vi "CRM-Config.vi"(6 "AI Channels":i32[](array[numeric]), 7 "Path":path, 8 "error in (no error)":errorcluster, 9 "Device Config":T1, 10 "Num AI pts":i32, 11 "Sampling Rate (Hz)":dbl=20000.0) -> (0 "error out":errorcluster, 1 "Magnitude array":dbl[](array[numeric]), 3 "Freq resol (Hz)":dbl)   [LabVIEW 2020]
uses:
  epl-vi-lib/PXI DAQ VIs/TDT VIs/Typedefs/TDT-Device Config.ctl
  epl-vi-lib/PXI DAQ VIs/TDT VIs/Typedefs/TDT-Output source.ctl
  epl-vi-lib/PXI DAQ VIs/TDT VIs/Typedefs/TDT-Device ID.ctl
  epl-vi-lib/PXI DAQ VIs/TDT VIs/Typedefs/TDT-Input source.ctl
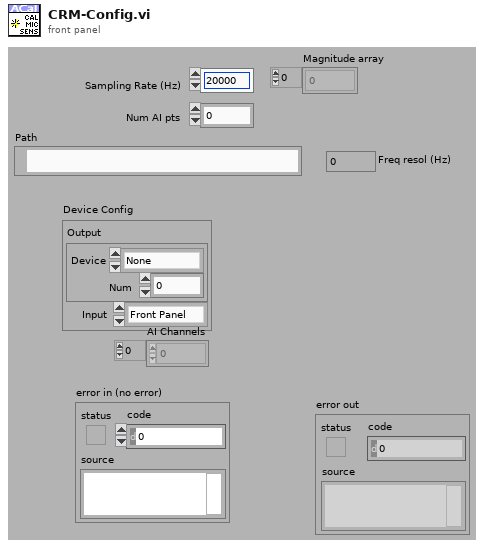
[diagram p1: front panel]
types:
  T1 = typedef "TDT-Device Config.ctl" = cluster{"Output":T2, "Input":T4}
  T2 = typedef "TDT-Output source.ctl" = cluster{"Device":T3, "Num":i32}
  T3 = typedef "TDT-Device ID.ctl" = enum16{"None", "PA5", "RP2", "RL2", "RA16", "RV8", "RX5", "RX6", "RX7", "RX8", "RZ2", "RZ5", "RZ6"}
  T4 = typedef "TDT-Input source.ctl" = enum16{"Front Panel", "RA4LI", "RA16LI"}
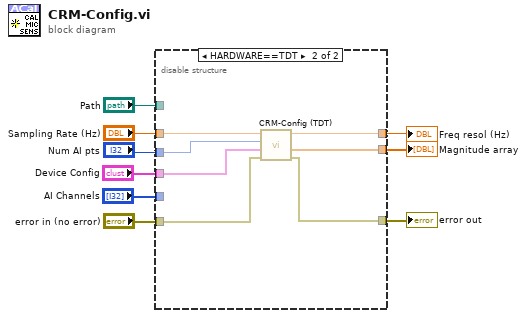
[diagram p0: block diagram]
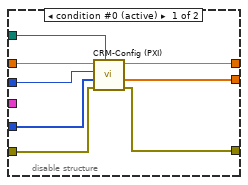
[diagram p2: hidden frame]
diagram:
  n1 = disable-structure shown="HARDWARE==TDT" {
    disable-tunnel: [w17 w24] -> w9
    disable-tunnel: "Num AI pts" -> [w16 w23]
    disable-tunnel: "Sampling Rate (Hz)" -> [w15 w22]
    disable-tunnel: [w14 w21] -> w6
    disable-tunnel: [w13 w20] -> w5
    disable-tunnel: "error in (no error)" -> [w12 w19]
    disable-tunnel: "Device Config" -> [_ w18]
    disable-tunnel: "AI Channels" -> [w11 _]
    disable-tunnel: "Path" -> [w10 _]
    frame condition #0 (active) {
      n2 = call "CRM-Config (PXI).vi"("Path"=w10, "error in (no error)"=w12, "AI Channels"=w11, "Num AI pts"=w16, "Sampling Rate (Hz)"=w15) -> ("error out"=w17:errorcluster, "Magnitude array"=w13:dbl[], "Freq resol (Hz)"=w14:dbl)  [unwired: 4 in]
    }
    frame condition #1 {
      n3 = call "CRM-Config (TDT).vi"("error in (no error)"=w19, "TDT"=w18, "Num AI pts"=w23, "Sampling Rate (Hz)"=w22) -> ("error out"=w24:errorcluster, "Magnitude array"=w20:dbl[], "Freq resol (Hz)"=w21:dbl)  [unwired: 5 in]
    }
  }
  "error out" <- w9
  "Freq resol (Hz)" <- w6
  "Magnitude array" <- w5
